vi "Pulse Measurements.vi"   [LabVIEW 2020, in "NI_MAPro.lvlib"]
doc: "Accepts a periodic waveform or an array of periodic waveforms and returns the <B>period</B>, <B>pulse duration</B> (pulse width), <B>duty cycle</B> (duty factor), and <B>pulse center</B> of a selected pulse and period. Wire data to the <B>signal in</B> input to determine the polymorphic instance to use or manually select the instance."
uses:
  NI_MAPro.lvlib
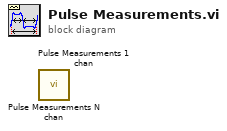
[diagram p0: block diagram]
diagram:
  n1 = call "Pulse Measurements N chan.vi"() -> ()  [unwired: 7 in, 5 out]
  n2 = call "Pulse Measurements 1 chan.vi"() -> ()  [unwired: 7 in, 5 out]
